vi "sonarSetLights.vi"(0 "error in":errorcluster, 2 "Lights":T1, 3 "node":string) -> (1 "error out":errorcluster)   [LabVIEW 2012]
uses:
  <userlib>/ROSforLV/ROS/Code/Console/Servers/ServerSubs/TopicDef.ctl
  <userlib>/ROSforLV/ROS/Code/SubVIs/_ROSDirection.ctl
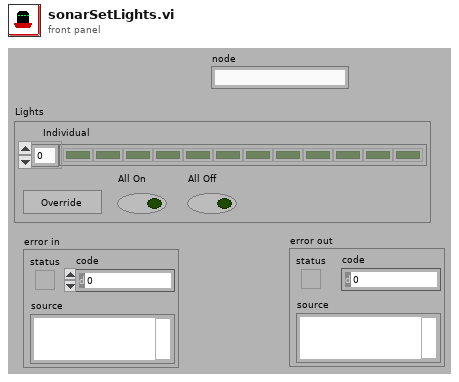
[diagram p1: front panel]
types:
  T1 = cluster{"Behavior":bool, "All On":bool, "All Off":bool, "Individual":bool[]}
  T2 = typedef "TopicDef.ctl" = cluster{"Topic":string, "Type":string, "Action":T3, "Update (ms)":u16, "write queue":u16}
  T3 = typedef "_ROSDirection.ctl" = enum16{"Node", "Publisher", "Subscriber", "Service Client"}
  T4 = typedef "_ROSControl.ctl" = cluster{"topic port":u16, "Node":string, "topic":string, "type":string, "node port":u16, "error ":errorcluster, "Direction":T3, "APIs":string[], "Update (ms)":u16, "write queue":u16}
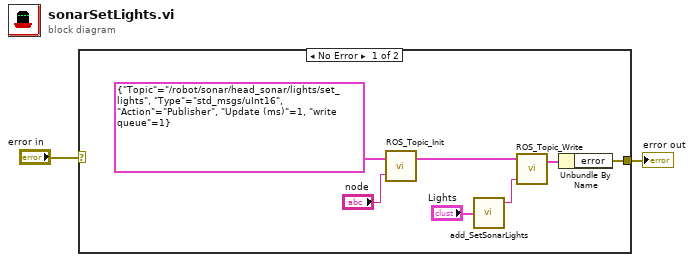
[diagram p0: block diagram]
diagram:
  n1 = case shown="No Error" "error in" {
    selector: "error in" -> [_ w10]
    tunnel: [w9 w10] -> w2
    frame No Error {
      n2 = call <userlib>:"ROS_Topic_Init.vi"("node"="node", "Definitions"=T2 {"Topic"="/robot/sonar/head_sonar/lights/set_lights", "Type"="std_msgs/uInt16", "Action"=enum."Publisher", "Update (ms)"=1, "write queue"=1}) -> ("ROS out"=w7:T4)  [unwired: 1 in]
      n3 = call <userlib>:"add_SetSonarLights.vi"("Lights"="Lights") -> ("msg out"=w4:string)  [unwired: 4 in]
      n4 = call <userlib>:"ROS_Topic_Write.vi"("Msg in"=w4, "ROS in"=w7) -> ("ROS out"=w6:T4)  [unwired: 2 in]
      n5 = Unbundle By Name(w6) -> ("error"=w9:errorcluster)
    }
    frame Error {
    }
  }
  "error out" <- w2
